vi "Add DPID.vi"(8 "error in (no error)":errorcluster, 11 "Node Ptr":u64 format="%.0x") -> (0 "error out":errorcluster)   [LabVIEW 2015, in "Diagnostics Addon System Explorer.lvlib"]
uses:
  Diagnostics Addon System Explorer.lvlib
  <vilib>/NI Veristand/Custom Device Tools/Custom Device Utility Library/Search Direction.ctl
  Types/FG Action.ctl
  Types/Exported DPID Parameters.ctl
  Shared/Types/DPID Parameters.ctl
  Shared/Types/DPID Periodic Rate.ctl
  SubVIs/ID FG.vi
  SubVIs/Get Signals.vi
  SubVIs/Type FG.vi
  SubVIs/Signal Parameters FG.vi
  Shared/SubVIs/GUID Lookup.vi
  <vilib>/NI Veristand/Custom Device API/NI VeriStand - Set Item Property.vi
  <vilib>/NI Veristand/Custom Device API/Set Item Property (U32).vi
  <vilib>/NI Veristand/Custom Device API/NI VeriStand - Get Item Property.vi
  <vilib>/NI Veristand/Custom Device API/Get Item Property (U32).vi
  <vilib>/NI Veristand/Custom Device API/Set Item Property (U32 Array).vi
  <vilib>/NI Veristand/Custom Device API/Get Item Property (U32 Array).vi
  <vilib>/NI Veristand/Custom Device Tools/Custom Device Utility Library/NI VeriStand - Search for Item by GUID.vi
  <vilib>/NI Veristand/Custom Device API/NI VeriStand - Get Item Data.vi
  <vilib>/NI Veristand/Custom Device API/Set Item Property (Double).vi
  <vilib>/NI Veristand/Custom Device API/Set Item Property (String).vi
  <vilib>/NI Veristand/Custom Device API/Get Item Property (Double).vi
  <vilib>/NI Veristand/Custom Device API/Get Item Property (String).vi
  <vilib>/NI Veristand/Custom Device API/NI VeriStand - Get Item Description.vi
  <vilib>/NI Veristand/Custom Device API/NI VeriStand - Get Custom Device Channel Data.vi
  <vilib>/NI Veristand/Custom Device Tools/Custom Device Utility Library/Custom Device Utility Library.lvlib
  Shared/Diagnostics Addon Shared.lvlib
  <vilib>/NI Veristand/Custom Device API/Custom Device API.lvlib
panel:
  in  "Tag":string
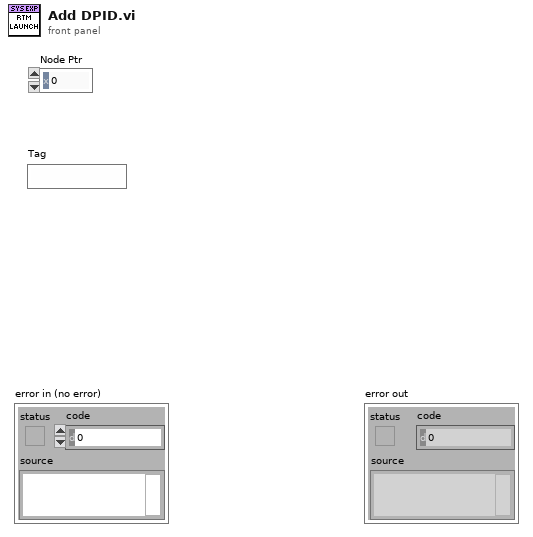
[diagram p1: front panel]
types:
  T1 = typedef "Custom Device Utility Library.lvlib/Search Direction.ctl" = enum16{"Down", "Up"}
  T2 = typedef "Custom Device API.lvlib/Custom Device Item Ref.ctl" = u64
  T3 = typedef "Diagnostics Addon System Explorer.lvlib/FG Action.ctl" = enum16{"Get", "Set"}
  T4 = typedef "Diagnostics Addon Shared.lvlib/DPID Parameters.ctl" = cluster{"DPID ID":u8, "Speed":T5, "PIDs":u16[]}
  T5 = typedef "Diagnostics Addon Shared.lvlib/DPID Periodic Rate.ctl" = enum16{"Slow", "Medium", "Fast"}
  T6 = typedef "Diagnostics Addon Shared.lvlib/Frame Parameters.ctl" = cluster{"Name":string, "Description":string, "ID":u32, "Type":T7, "Signals":T8[]}
  T7 = typedef "Diagnostics Addon Shared.lvlib/MessageType Selector.ctl" = enum16{"DID", "PID", "CPID", "Write Memory", "Read Memory", "DTC Control", "IO Cmd", "IO Resp", "Routine Start Cmd", "Routine Start Resp", "Routine Status Cmd", "Routine Status Resp", "Routine Stop Cmd", "Routine Stop Resp"}
  T8 = typedef "Diagnostics Addon Shared.lvlib/Signal Parameters.ctl" = cluster{"Start Bit":u8, "Length":u8, "Scaling Factor":dbl, "Scaling Offset":dbl, "Minimum":dbl, "Maximum":dbl, "Data Type":u32, "Byte Order":u32, "Default Value":dbl, "Name":string, "Units":string, "Description":string}
  T9 = typedef "Diagnostics Addon System Explorer.lvlib/Exported DPID Parameters.ctl" = cluster{"Name":string, "Description":string, "DPID":T4}
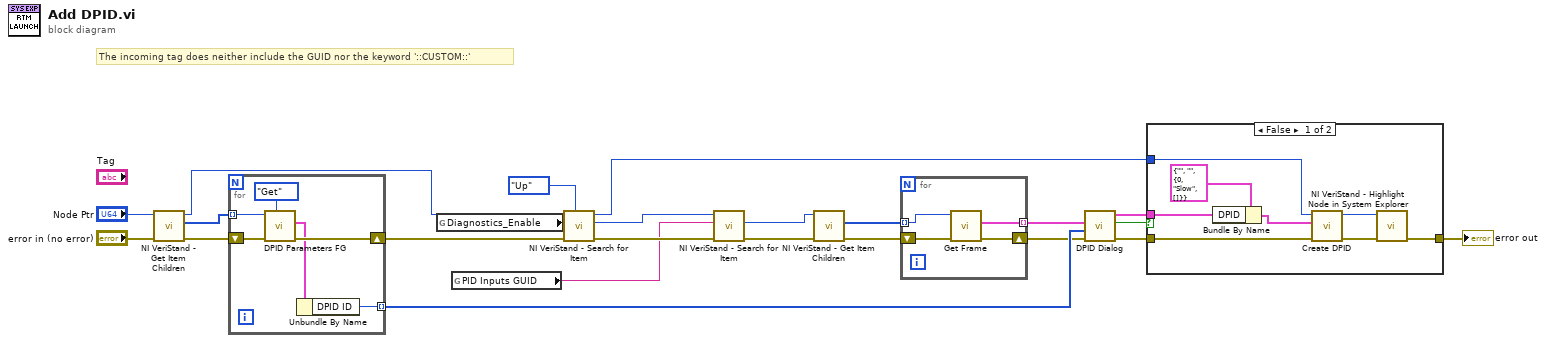
[diagram p0: block diagram]
diagram:
  # "The incoming tag does neither include the GUID nor the keyword '::CUSTOM::'"
  n1 = call <vilib>:"NI VeriStand - Get Item Children.vi"("error in (no error)"="error in (no error)", "Item Ref in"="Node Ptr") -> ("error out"=w12:errorcluster, "Child Refs"=w13:T2[], "Item Ref out"=w14:T2)  [unwired: 6 in, 1 out]
  n2 = for {
    tunnel: w13 -> [w29] mode=indexing
    shift-right: [w27] -> w11
    shift-left: w12 -> [w28]
    tunnel: [w25] -> w10 mode=indexing
    n3 = call "DPID Parameters FG.vi"("Action"=FG_Action."Get", "error in (no error)"=w28, "Device Item Ref in"=w29) -> ("error out"=w27:errorcluster, "DPID"=w26:T4)  [unwired: 6 in, 1 out]
    n4 = Unbundle By Name(w26) -> ("DPID ID"=w25:u8)
  }
  n5 = global read "GUID Lookup.vi" "Diagnostics_Enable"() -> (w23:string)
  n6 = global read "GUID Lookup.vi" "PID Inputs GUID"() -> (w19:string)
  n7 = call-poly <vilib>:"NI VeriStand - Search for Item.vi"("Direction (Down)"=Search_Direction."Up", "error in"=w11, "Item GUID"=w23, "Section Ref in"=w14) -> ("error out"=w20:errorcluster, "Item Ref"=w21:T2, "Section Ref out"=w5:T2)  [unwired: 4 in, 1 out]
  n8 = call-poly <vilib>:"NI VeriStand - Search for Item.vi"("error in"=w20, "Item GUID"=w19, "Section Ref in"=w21) -> ("error out"=w18:errorcluster, "Item Ref"=w17:T2)  [unwired: 5 in, 2 out]
  n9 = call <vilib>:"NI VeriStand - Get Item Children.vi"("error in (no error)"=w18, "Item Ref in"=w17) -> ("error out"=w2:errorcluster, "Child Refs"=w3:T2[])  [unwired: 6 in, 2 out]
  n10 = for {
    tunnel: w3 -> [w33] mode=indexing
    tunnel: [w30] -> w4 mode=indexing
    shift-right: [w31] -> w1
    shift-left: w2 -> [w32]
    n11 = call "Get Frame.vi"("error in (no error)"=w32, "Item Ref in"=w33) -> ("error out"=w31:errorcluster, "PID In"=w30:T6)  [unwired: 7 in, 1 out]
  }
  n12 = call "DPID Dialog.vi"("error in (no error)"=w1, "Existing DPIDs"=w10, "Existing PIDs"=w4) -> ("error out"=w7:errorcluster, "Cancel PID?"=w9:bool, "DPID"=w8:T4)  [unwired: 6 in]
  n13 = case shown="False" w9 {
    tunnel: w8 -> [w39 _]
    tunnel: w7 -> [w41 w42]
    tunnel: [w35 w42] -> w6
    tunnel: w5 -> [w40 _]
    frame False {
      n14 = Bundle By Name(cluster=T9 {"Name"="", "Description"="", "DPID"={"DPID ID"=0, "Speed"=enum."Slow", "PIDs"=[]}} ("DPID"), "DPID"=w39) -> (w37:T9)
      n15 = call "Create DPID.vi"("error in (no error)"=w41, "DPID"=w37, "Section Ptr"=w40) -> ("error out"=w36:errorcluster, "Parent Ref out"=w34:T2)  [unwired: 7 in]
      n16 = call <vilib>:"NI VeriStand - Highlight Node in System Explorer.vi"("error in (no error)"=w36, "Item Ref in"=w34) -> ("error out"=w35:errorcluster)  [unwired: 8 in, 1 out]
    }
    frame True {
    }
  }
  "error out" <- w6
